vi "MOPX2 Crossover.vi"(6 "Operation Selection":T1, 8 "error in (no error)":errorcluster, 9 "Parent 2 Schedule":u16[](array[numeric]), 10 "Parent 1 Schedule":u16[](array[numeric]), 11 "OSSP_Problem In":refnum<class "OSSP_Problem.lvclass">) -> (0 "error out":errorcluster, 1 "Child 2":T2, 2 "Child 1":T2, 3 "OSSP_Problem out":refnum<class "OSSP_Problem.lvclass">)   [LabVIEW 2013, in "GA.lvclass"]
uses:
  GA.lvclass
  OSSP_Problem.lvclass
  Controls/Solution_GA.ctl
  Controls/MPOX2 Operation Selection Rule.ctl
panel:
  out "Child 2 Schedule":u16[](array[numeric])
  out "Child 1 Schedule":u16[](array[numeric])
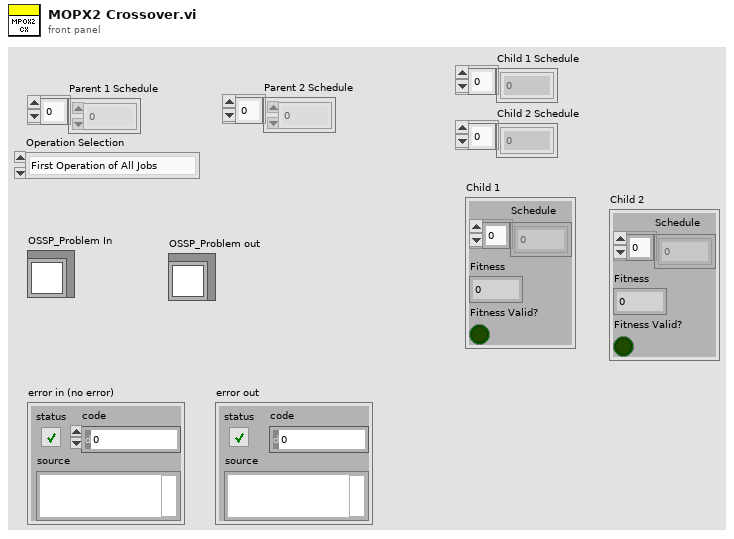
[diagram p1: front panel]
types:
  T1 = typedef "GA.lvclass/MPOX2 Operation Selection Rule.ctl" = enum16{"First Operation of All Jobs", "Random"}
  T2 = typedef "Solution_GA.ctl" = cluster{"Schedule":u16[], "Fitness":u16, "Fitness Valid?":bool}
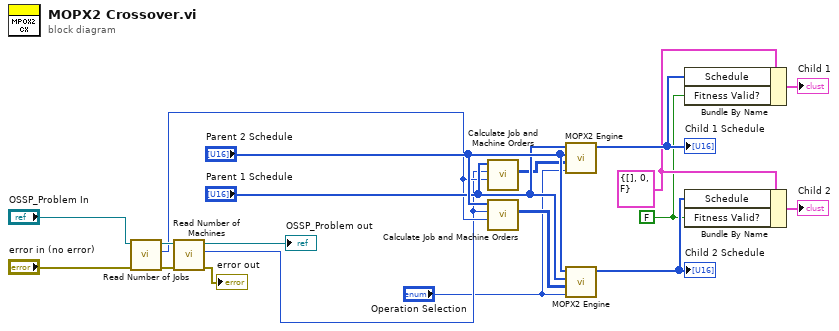
[diagram p0: block diagram]
diagram:
  w6 = FALSE ("Fitness Valid?")
  w7 = T2 {"Schedule"=[], "Fitness"=0, "Fitness Valid?"=FALSE} ("Child 2")
  n1 = call-dynamic "Read Number of Jobs.vi"("error in (no error)"="error in (no error)", "OSSP_Problem in"="OSSP_Problem In") -> ("error out"=w16:errorcluster, "Number of Jobs"=w14:i32, "OSSP_Problem out"=w15:refnum<class "OSSP_Problem.lvclass">)  [unwired: 7 in]
  n2 = call-dynamic "Read Number of Machines.vi"("error in (no error)"=w16, "OSSP_Problem in"=w15) -> ("error out"=→"error out":errorcluster, "Number of Machines"=w13:i32, "OSSP_Problem out"=→"OSSP_Problem out":refnum<class "OSSP_Problem.lvclass">)  [unwired: 7 in]
  n3 = call "Calculate Job and Machine Orders.vi"("Number of Jobs"=w14, "Number of Machines"=w13, "Schedule"="Parent 1 Schedule") -> ("MO4J"=w10:u16[][])  [unwired: 7 in, 1 out]
  n4 = call "Calculate Job and Machine Orders.vi"("Number of Jobs"=w14, "Number of Machines"=w13, "Schedule"="Parent 2 Schedule") -> ("MO4J"=w9:u16[][])  [unwired: 7 in, 1 out]
  n5 = call "MOPX2 Engine.vi"("Operation Selection"="Operation Selection", "Main Parent  MO4J"=w10, "Secondary Parent Schedule"="Parent 2 Schedule", "Main Parent Schedule"="Parent 1 Schedule") -> ("Child Schedule"=w12:u16[])  [unwired: 7 in]
  "Child 1 Schedule" <- w12
  n6 = call "MOPX2 Engine.vi"("Operation Selection"="Operation Selection", "Main Parent  MO4J"=w9, "Secondary Parent Schedule"="Parent 1 Schedule", "Main Parent Schedule"="Parent 2 Schedule") -> ("Child Schedule"=w11:u16[])  [unwired: 7 in]
  "Child 2 Schedule" <- w11
  n7 = Bundle By Name(cluster=w7, "Schedule"=w12, "Fitness Valid?"=w6) -> (→"Child 1":T2)
  n8 = Bundle By Name(cluster=w7, "Schedule"=w11, "Fitness Valid?"=w6) -> (→"Child 2":T2)
